vi "StringToBoolean.vi"(1 "String":string) -> (0 "Output":bool)   [LabVIEW 2019]
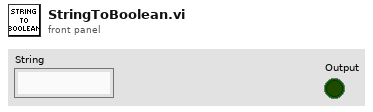
[diagram p1: front panel]
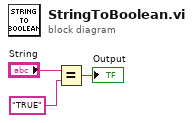
[diagram p0: block diagram]
diagram:
  n1 = Equal?(x="String", y="TRUE") -> (x = y?=→"Output":bool)
